vi "DB select data(cmd).vi"(8 "error in (no error)":errorcluster caption="错误输入（无错误）", 9 "Select cmd":string, 10 "Tabe":string, 11 "Connncet State":T1) -> (0 "error out":errorcluster caption="错误输出", 1 "state":bool, 2 "data":variant[][](array[variant]), 3 "Connncet State out":T1)   [LabVIEW 2014]
uses:
  <vilib>/addons/database/NI_Database_API.lvlib
  Ctr/Constr.ctl
  <vilib>/addons/database/Connection.llb/Conn ObjectReference.ctl
  Ctr/Conneect State.ctl
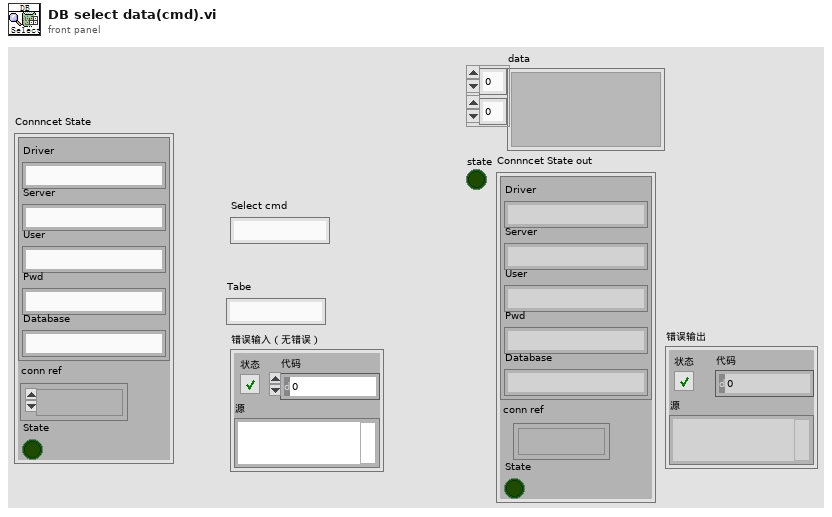
[diagram p1: front panel]
types:
  T1 = typedef "Conneect State.ctl" = cluster{"Constr":T2, "conn ref":T3, "State":bool}
  T2 = typedef "Constr.ctl" = cluster{"Driver":string, "Server":string, "User":string, "Pwd":string, "Database":string}
  T3 = typedef "NI_Database_API.lvlib/Conn ObjectReference.ctl" = refnum<k1>
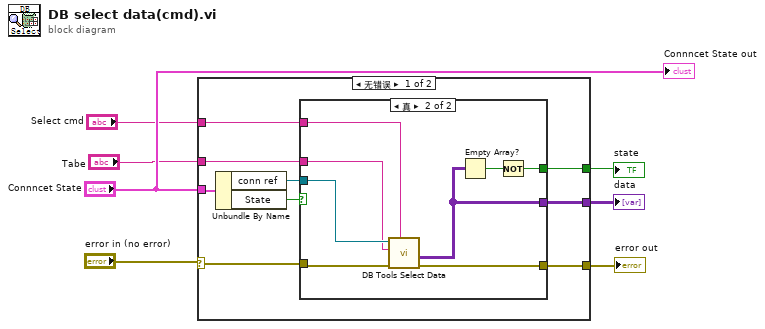
[diagram p0: block diagram]
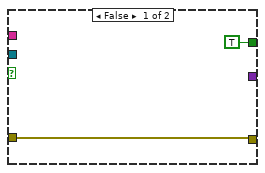
[diagram p2: hidden frame]
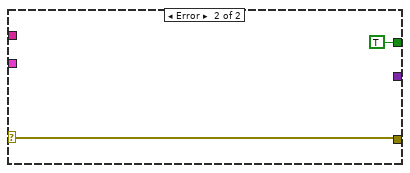
[diagram p3: hidden frame]
diagram:
  n1 = case shown="无错误" "error in (no error)" {
    selector: "error in (no error)" -> [w14 w28]
    tunnel: "Connncet State" -> [w16 _]
    tunnel: "Tabe" -> [w12 _]
    tunnel: "Select cmd" -> [w11 _]
    tunnel: [w10 w28] -> w3
    tunnel: [w9 _] -> w2
    tunnel: [w8 TRUE] -> w1
    frame No Error {
      n2 = Unbundle By Name(w16) -> ("conn ref"=w13:T3, "State"=w15:bool)
      n3 = case shown="真" w15 {
        tunnel: w14 -> [w18 w26]
        tunnel: w13 -> [_ w25]
        tunnel: w12 -> [_ w24]
        tunnel: w11 -> [_ w23]
        tunnel: [w18 w22] -> w10
        tunnel: [_ w21] -> w9
        tunnel: [TRUE w19] -> w8
        frame False {
        }
        frame True {
          n4 = call <vilib>:"DB Tools Select Data.vi"("condition"=w23, "error in (no error)"=w26, "table"=w24, "connection reference"=w25) -> ("error out"=w22:errorcluster, "data"=w21:variant[][])  [unwired: 2 in, 1 out]
          n5 = Empty Array?(array=w21) -> (empty?=w20:bool)
          n6 = Not(x=w20) -> (.not. x?=w19:bool)
        }
      }
    }
    frame Error {
    }
  }
  "error out" <- w3
  "data" <- w2
  "state" <- w1
  "Connncet State out" <- "Connncet State"
